vi "test.vi"() -> ()   [LabVIEW 2010]
panel:
  in  "清0":bool
  in  "读入":bool
  out "数值 3":u64
  in  "数值 2":u64
  out "开始时间":dbl format="%#.0f"
  out "结束?":bool
  in  "停止":bool
  in  "数值":dbl
  in  "开始":bool
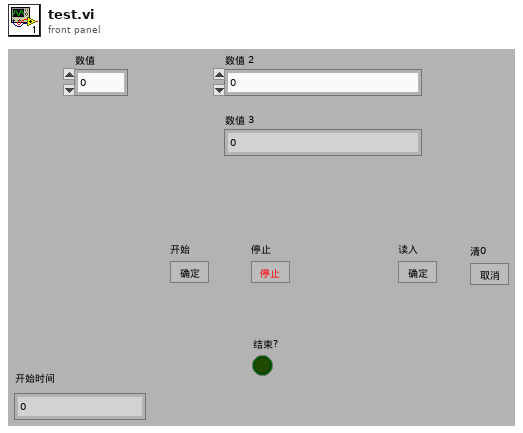
[diagram p1: front panel]
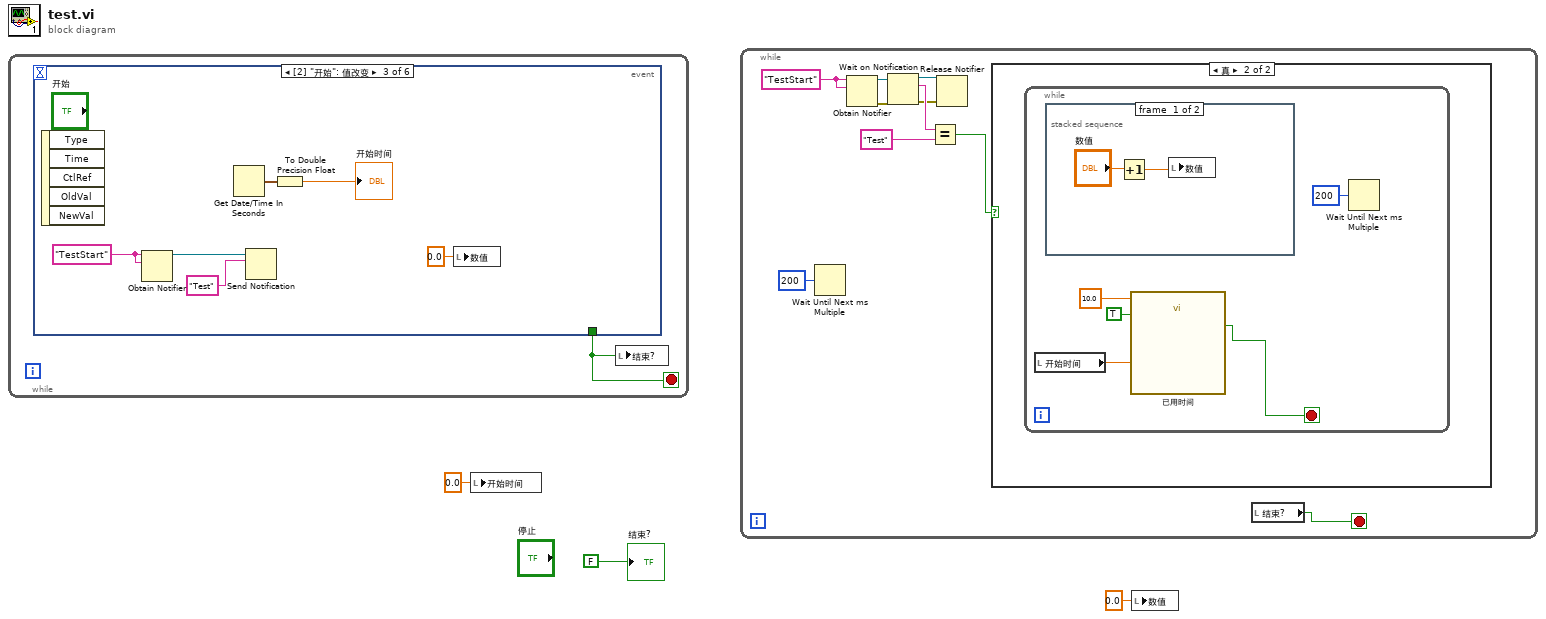
[diagram p0: block diagram]
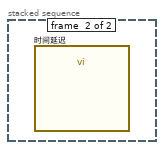
[diagram p3: hidden frame]
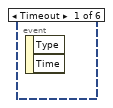
[diagram p4: hidden frame]
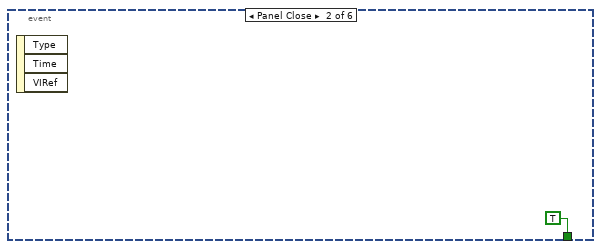
[diagram p5: hidden frame]
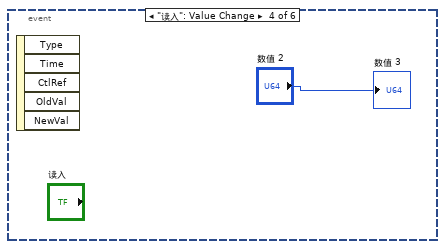
[diagram p6: hidden frame]
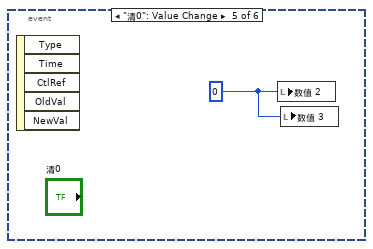
[diagram p7: hidden frame]
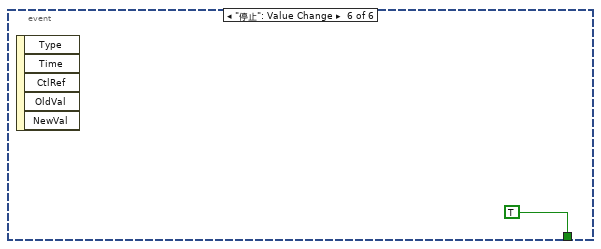
[diagram p8: hidden frame]
diagram:
  n1 = while {
    stop <- w4 stop-if-true
    n2 = event shown="[2] \"开始\": 值改变" {
      selector: _ -> [_ _ _ _ _ _]
      dyn-events: _ -> [_ _ _ _ _ _]
      timeout: _ -> [_ _ _ _ _ _]
      tunnel: [_ TRUE _ _ _ TRUE] -> w4
      event Timeout {
        n3 = event-data() -> ()  [unwired: 1 in, 2 out]
      }
      event Panel Close {
        n4 = event-data() -> ()  [unwired: 1 in, 3 out]
      }
      event "开始": Value Change {
        w7 = "TestStart" ("名称（未命名）")
        n5 = event-data() -> ()  [unwired: 1 in, 5 out]
        n6 = Obtain Notifier(name (unnamed)=w7, notification data type=w7) -> (notifier out=w6:refnum<notifier>)  [unwired: 2 in, 2 out]
        n7 = Get Date/Time In Seconds() -> (seconds since 1Jan1904=w10:timestamp)
        n8 = Send Notification(notification="Test" ("通知"), notifier=w6) -> ()  [unwired: 1 in, 2 out]
        n9 = To Double Precision Float(number=w10) -> (double precision float=→"开始时间":dbl)
        n10 = local write "数值"(0.0 ("数值")) -> ()
      }
      event "读入": Value Change {
        n11 = event-data() -> ()  [unwired: 1 in, 5 out]
        "数值 3" <- "数值 2"
      }
      event "清0": Value Change {
        w13 = 0 ("数值 2")
        n12 = event-data() -> ()  [unwired: 1 in, 5 out]
        n13 = local write "数值 2"(w13) -> ()
        n14 = local write "数值 3"(w13) -> ()
      }
      event "停止": Value Change {
        n15 = event-data() -> ()  [unwired: 1 in, 5 out]
      }
    }
    n16 = local write "结束?"(w4) -> ()
  }
  n17 = local write "开始时间"(0.0 ("开始时间")) -> ()
  n18 = while {
    stop <- w15 stop-if-true
    w18 = "TestStart" ("名称（未命名）")
    n19 = Wait Until Next ms Multiple(millisecond multiple=u32 200 ("毫秒倍数")) -> ()  [unwired: 1 out]
    n20 = Obtain Notifier(name (unnamed)=w18, notification data type=w18) -> (notifier out=w20:refnum<notifier>, error out=w21:errorcluster)  [unwired: 2 in, 1 out]
    n21 = Wait on Notification(notifier=w20, error in (no error)=w21) -> (notifier out=w22:refnum<notifier>, notification=w24:string, error out=w23:errorcluster)  [unwired: 2 in, 1 out]
    n22 = Equal?(x=w24, y="Test" ("通知")) -> (x = y?=w17:bool)
    n23 = Release Notifier(notifier=w22, error in (no error)=w23) -> ()  [unwired: 1 in, 3 out]
    n24 = case shown="真" w17 {
      frame False {
      }
      frame True {
        n25 = while {
          stop <- w28 stop-if-true
          n26 = local read "开始时间"() -> (w29:dbl)
          n27 = stacked-sequence {
            frame #0 {
              n28 = Increment(x="数值") -> (x+1=w30:dbl)
              n29 = local write "数值"(w30) -> ()
            }
            frame #1 {
              n30 = call "时间延迟"() -> ()  [unwired: 11 in, 1 out]
            }
          }
          n31 = call "已用时间"("Time Target (s)"=10.0, "Reset"=TRUE, "Set Start Time (s)"=w29) -> ("Time has Elapsed"=w28:bool)  [unwired: 9 in, 7 out]
          n32 = Wait Until Next ms Multiple(millisecond multiple=u32 200 ("毫秒倍数")) -> ()  [unwired: 1 out]
        }
      }
    }
    n33 = local read "结束?"() -> (w15:bool)
  }
  n34 = local write "数值"(0.0 ("数值")) -> ()
  "结束?" <- FALSE
